vi "Email and Text Notification.vi"(0 "Message Main Body":string="Error occurred") -> ()   [LabVIEW 2013]
panel:
  in  "Attachment - Optional":path
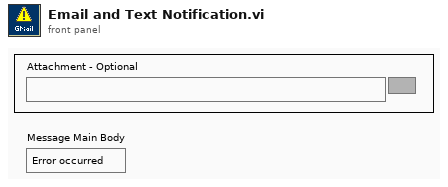
[diagram p1: front panel]
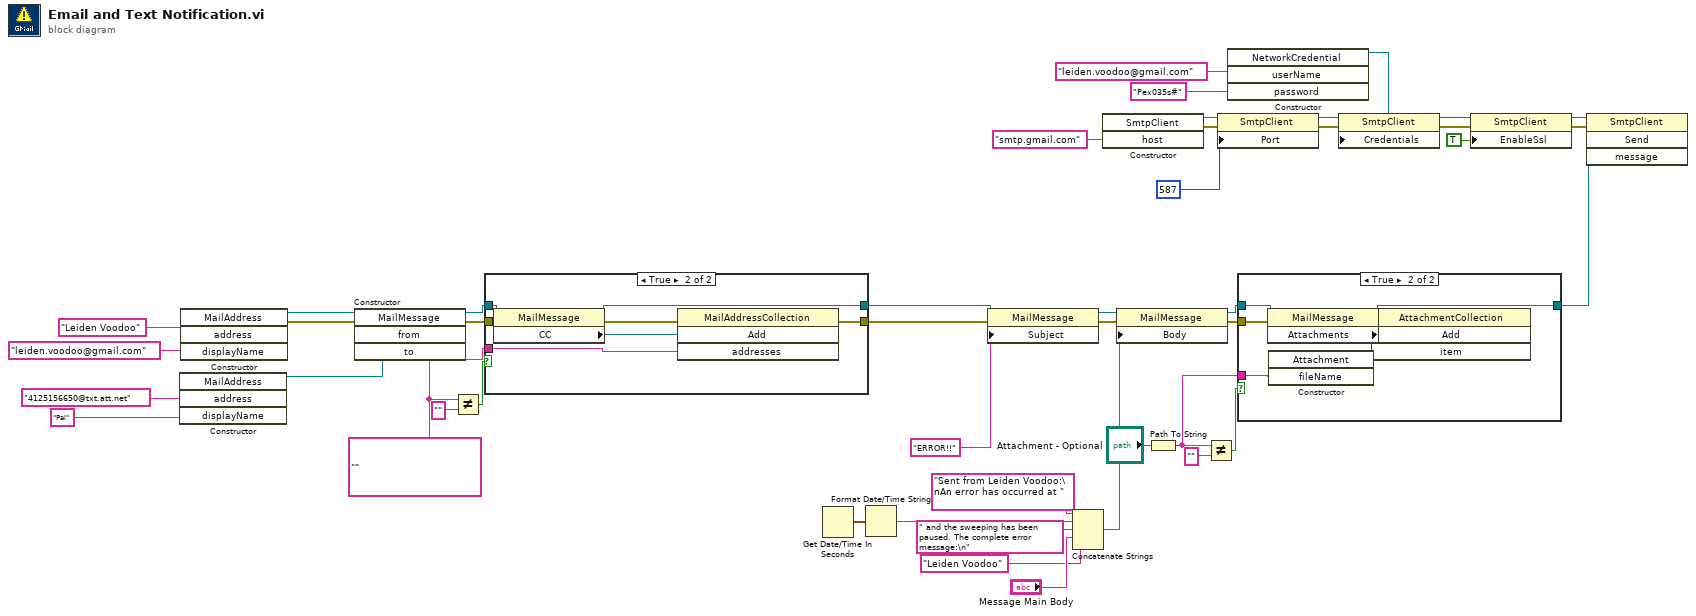
[diagram p0: block diagram]
diagram:
  w17 = "" ("CC - Optional")
  n1 = constructor class="MailAddress"("address"="4125156650@txt.att.net" ("Recipient's Email Address"), "displayName"="Pai" ("Recipient's Name")) -> (reference out=w45:refnum<k24>)  [unwired: 3 in, 4 out]
  n2 = constructor class="MailAddress"("address"="leiden.voodoo@gmail.com" ("Sender's Email Address (eg: LabVIEW@gmail.com)"), "displayName"="Leiden Voodoo" ("Sender's Name")) -> (reference out=w44:refnum<k24>, error out=w9:errorcluster)  [unwired: 3 in, 3 out]
  n3 = constructor class="MailMessage"(error in=w9, "from"=w44, "to"=w45) -> (reference out=w16:refnum<k24>, error out=w15:errorcluster)  [unwired: 2 in, 3 out]
  n4 = Not Equal?(x=w17, y="") -> (x != y?=w18:bool)
  n5 = case shown="True" w18 {
    tunnel: w17 -> [_ w52]
    tunnel: w16 -> [w47 w51]
    tunnel: w15 -> [w46 w50]
    tunnel: [w47 w49] -> w14
    tunnel: [w46 w48] -> w13
    frame False {
    }
    frame True {
      n6 = property class="MailMessage"(reference=w51, error in=w50) -> (reference out=w49:refnum<k24>, error out=w54:errorcluster, "CC"=w53:refnum<k24>)
      n7 = invoke class="MailAddressCollection" method="Add"(reference=w53, error in=w54, "addresses"=w52) -> (error out=w48:errorcluster)  [unwired: 1 in, 3 out]
    }
  }
  n8 = Get Date/Time In Seconds() -> (seconds since 1Jan1904=w3:timestamp)
  n9 = Format Date/Time String(seconds (now)=w3) -> (date/time string=w2:string)  [unwired: 2 in]
  n10 = property class="MailMessage"(reference=w14, error in=w13, "Subject"="ERROR!!") -> (reference out=w36:refnum<k24>, error out=w43:errorcluster)
  n11 = Concatenate Strings("Sent from Leiden Voodoo:\nAn error has occurred at " ("string"), w2, " and the sweeping has been paused. The complete error message:\n" ("string"), "Message Main Body", "Leiden Voodoo" ("string")) -> (w6:string)
  n12 = constructor class="SmtpClient"("host"="smtp.gmail.com" ("Outgoing Mail Server (SMTP)")) -> (reference out=w30:refnum<k24>, error out=w27:errorcluster)  [unwired: 3 in, 2 out]
  n13 = property class="MailMessage"(reference=w36, error in=w43, "Body"=w6) -> (reference out=w24:refnum<k24>, error out=w8:errorcluster)
  n14 = Path To String(path="Attachment - Optional") -> (string=w20:string)
  n15 = Not Equal?(x=w20, y="") -> (x != y?=w21:bool)
  n16 = property class="SmtpClient"(reference=w30, error in=w27, "Port"=587) -> (reference out=w29:refnum<k24>, error out=w26:errorcluster)
  n17 = constructor class="NetworkCredential"("userName"="leiden.voodoo@gmail.com" ("GMAIL Account User ID"), "password"="Pex035s#" ("GMAIL Account Password")) -> (reference out=w31:refnum<k24>)  [unwired: 3 in, 4 out]
  n18 = case shown="True" w21 {
    tunnel: w24 -> [w55 w59]
    tunnel: [w55 w58] -> w12
    tunnel: w20 -> [_ w57]
    tunnel: w8 -> [_ w56]
    frame False {
    }
    frame True {
      n19 = property class="MailMessage"(reference=w59, error in=w56) -> (reference out=w58:refnum<k24>, error out=w62:errorcluster, "Attachments"=w60:refnum<k24>)
      n20 = constructor class="Attachment"("fileName"=w57) -> (reference out=w61:refnum<k24>)  [unwired: 3 in, 3 out]
      n21 = invoke class="AttachmentCollection" method="Add"(reference=w60, error in=w62, "item"=w61) -> ()  [unwired: 1 in, 4 out]
    }
  }
  n22 = property class="SmtpClient"(reference=w29, error in=w26, "Credentials"=w31) -> (reference out=w28:refnum<k24>, error out=w25:errorcluster)
  n23 = property class="SmtpClient"(reference=w28, error in=w25, "EnableSsl"=TRUE ("Enable SSL")) -> (reference out=w10:refnum<k24>, error out=w11:errorcluster)
  n24 = invoke class="SmtpClient" method="Send"(reference=w10, error in=w11, "message"=w12) -> ()  [unwired: 1 in, 4 out]
